vi "SSC Digital Wait Until Done.vi"(0 "Digital SSC in":T1[](array[typedef]), 7 "timeout (s)":dbl=10.0, 11 "error in":errorcluster) -> (4 "Digital SSC out":T1[](array[typedef]), 15 "error out":errorcluster)   [LabVIEW 2020]
doc: "Waits until the pattern burst has completed or the timeout has expired on the specified pin(s) or pin group(s)."
uses:
  SSC Digital.ctl
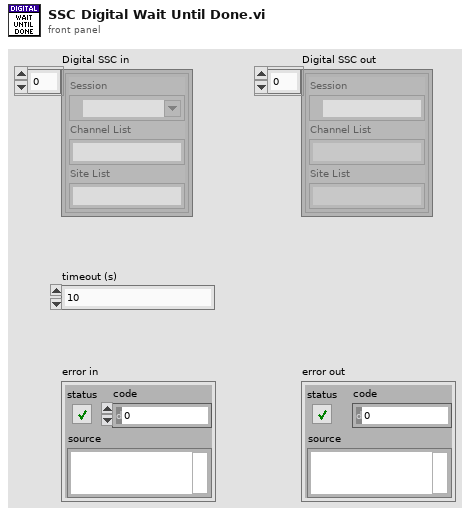
[diagram p1: front panel]
types:
  T1 = typedef "SSC Digital.ctl" = cluster{"Session":refnum<k15>, "Channel List":string, "Site List":string}
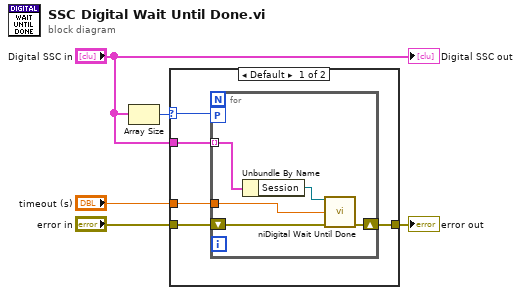
[diagram p0: block diagram]
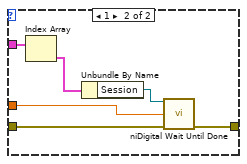
[diagram p2: hidden frame]
diagram:
  n1 = Array Size(array="Digital SSC in") -> (size(s)=w3:i32)
  n2 = case shown="Default" w3 {
    selector: w3 -> [w8 _]
    tunnel: "error in" -> [w10 w21]
    tunnel: [w9 w20] -> w4
    tunnel: "Digital SSC in" -> [w7 w19]
    tunnel: "timeout (s)" -> [w6 w18]
    frame Default {
      n3 = for {
        tunnel: w7 -> [w15] mode=indexing
        workers-P: w8 -> [_]
        shift-right: [w13] -> w9
        shift-left: w10 -> [w14]
        tunnel: w6 -> [w11]
        n4 = Unbundle By Name(w15) -> ("Session"=w12:refnum<k15>)
        n5 = call <instrlib>:"niDigital Wait Until Done.vi"("instrument handle"=w12, "timeout (s)"=w11, "error in"=w14) -> ("error out"=w13:errorcluster)  [unwired: 11 in, 1 out]
      }
    }
    frame 1 {
      n6 = Index Array(array=w19) -> (element=w16:T1)  [unwired: 1 in]
      n7 = Unbundle By Name(w16) -> ("Session"=w17:refnum<k15>)
      n8 = call <instrlib>:"niDigital Wait Until Done.vi"("instrument handle"=w17, "timeout (s)"=w18, "error in"=w21) -> ("error out"=w20:errorcluster)  [unwired: 11 in, 1 out]
    }
  }
  "error out" <- w4
  "Digital SSC out" <- "Digital SSC in"
